vi "ExtractCamNames.vi"(10 "filenames":string[](array[string]), 11 "name":string) -> (1 "CamNames":string[](array[string]))   [LabVIEW 2022 SP3]
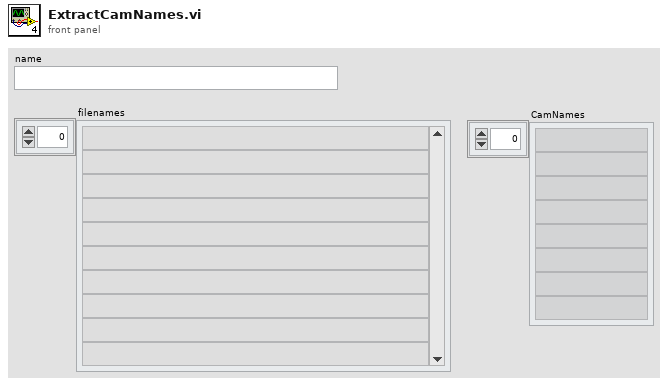
[diagram p1: front panel]
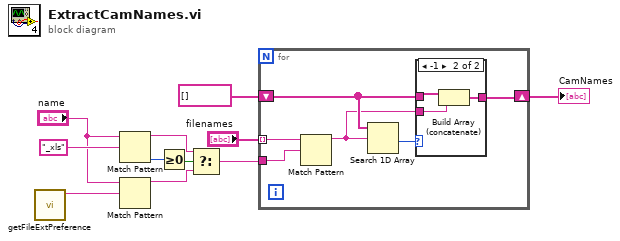
[diagram p0: block diagram]
diagram:
  n1 = call "getFileExtPreference.vi"() -> ("Suffix to add"=w6:string)  [unwired: 11 in]
  n2 = Match Pattern(string="name", regular expression="_xls") -> (before substring=w2:string, offset past match=w5:i32)  [unwired: 1 in, 2 out]
  n3 = Match Pattern(string="name", regular expression=w6) -> (before substring=w3:string)  [unwired: 1 in, 3 out]
  n4 = Greater Or Equal To 0?(x=w5) -> (x >= 0?=w4:bool)
  n5 = Select(t=w2, s=w4, f=w3) -> (s? t:f=w1:string)
  n6 = for {
    tunnel: "filenames" -> [w17] mode=indexing
    tunnel: w1 -> [w16]
    shift-right: [w12] -> w9
    shift-left: string[] [] -> [w14]
    n7 = Match Pattern(string=w17, regular expression=w16) -> (before substring=w13:string)  [unwired: 1 in, 3 out]
    n8 = Search 1D Array(1D array=w14, element=w13) -> (index of element=w15:i32)  [unwired: 1 in]
    n9 = case shown="-1" w15 {
      tunnel: w14 -> [w18 w21]
      tunnel: w13 -> [_ w20]
      tunnel: [w18 w19] -> w12
      frame 0, Default {
      }
      frame -1 {
        n10 = Build Array (concatenate)(w21, w20) -> (w19:string[])
      }
    }
  }
  "CamNames" <- w9
